vi "Popup.vi"(8 "error in (no error)":errorcluster, 9 "Panel":refnum<class "Panel.lvclass">, 10 "String in":string, 11 "String Data Type in":refnum<class "String Data Type.lvclass">) -> (0 "error out":errorcluster, 2 "String out":string, 3 "String Data Type out":refnum<class "String Data Type.lvclass">)   [LabVIEW 2018, in "String Data Type.lvclass"]
uses:
  String Data Type.lvclass
  <vilib>/MGI/Panel Manager/Panel/Panel/Panel.lvclass
  <vilib>/Utility/miscctls.llb/LVSelectionTypeDef.ctl
  String Data Type.lvclass/String Data Type.ctl
panel:
  in  "String":string
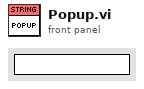
[diagram p1: front panel]
types:
  T1 = typedef "LVSelectionTypeDef.ctl" = cluster{"Selection Start":u32, "Selection End":u32}
  T2 = typedef "String Data Type.lvclass/Display Style Enum.ctl" = enum16{"Normal", "'\\' Codes", "Hex"}
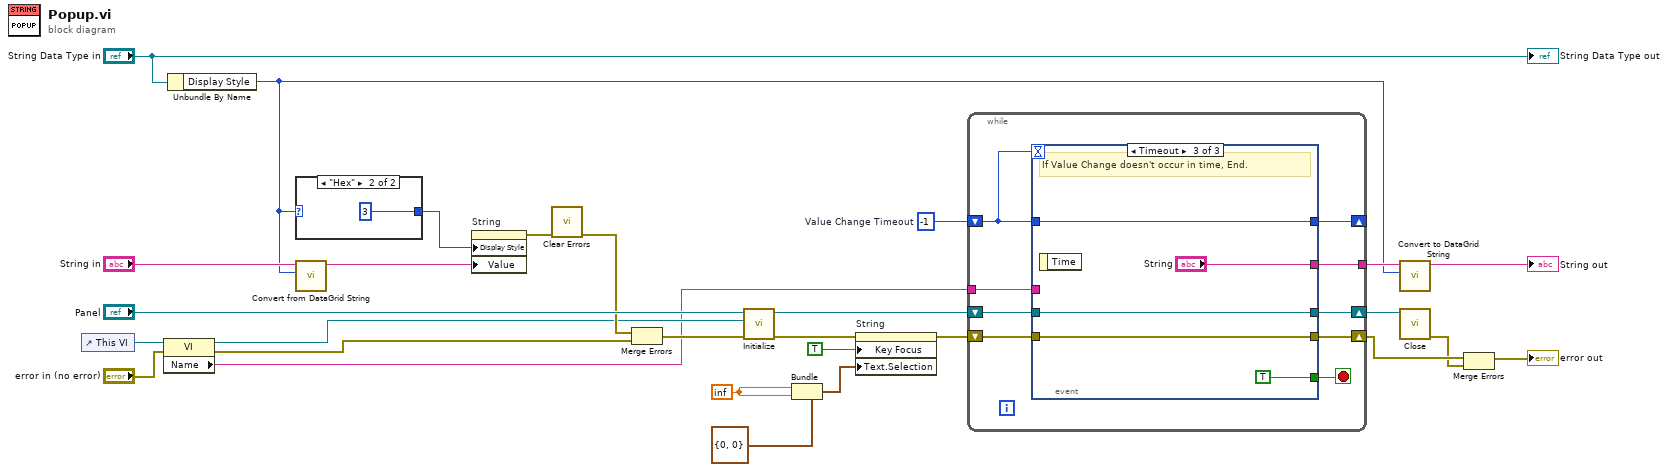
[diagram p0: block diagram]
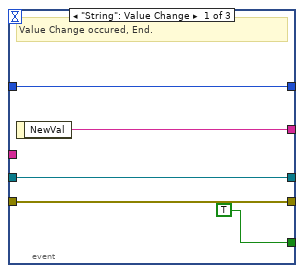
[diagram p3: hidden frame]
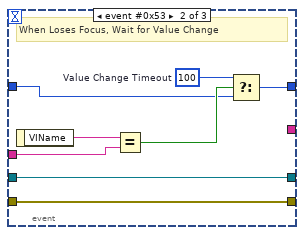
[diagram p4: hidden frame]
diagram:
  w9 = inf
  w14 = -1  # Value Change Timeout
  n1 = control-ref of="This VI"() -> (w20:refnum<vi>)
  n2 = property class="VI"(reference=w20, error in="error in (no error)") -> (reference out=w19:refnum<vi>, error out=w15:errorcluster, "Name"=w17:string)
  n3 = Unbundle By Name("String Data Type in") -> ("Display Style"=w2:T2)
  n4 = case shown="\"Hex\"" w2 {
    selector: w2 -> [w29 _]
    tunnel: [w29 u32 3] -> w1
    frame "Normal", "'\\' Codes" {
    }
    frame "Hex" {
    }
  }
  n5 = call "Convert from DataGrid String.vi"("Display Style"=w2, "DataGrid String in"="String in") -> ("Popup String out"=w6:string)  [unwired: 9 in]
  n6 = property on="String" class="Str"("Display Style"=w1, "Value"=w6) -> (error out=w22:errorcluster)  [unwired: 2 in, 1 out]
  n7 = call <vilib>:"Clear Errors.vi"("error in (no error)"=w22) -> ("error out"=w21:errorcluster)  [unwired: 5 in, 1 out]
  n8 = Merge Errors(w21, w15) -> (w18:errorcluster)
  n9 = call <vilib>:"Initialize.vi"("error in (no error)"=w18, "VI Refnum"=w19, "Panel In"="Panel") -> ("error out"=w12:errorcluster, "Panel Out"=w27:refnum<class "Panel.lvclass">)  [unwired: 6 in, 1 out]
  n10 = Bundle(cluster=T1 {"Selection Start"=0, "Selection End"=0} ("Text.Selection"), "Selection Start"=w9, "Selection End"=w9) -> (w8:T1)
  n11 = property on="String" class="Str"(error in=w12, "Key Focus"=TRUE, "Text.Selection"=w8) -> (error out=w11:errorcluster)  [unwired: 1 in, 1 out]
  n12 = while {
    shift-right: [w39] -> w25
    shift-left: w11 -> [w38]
    shift-right: [w36] -> w26
    shift-left: w27 -> [w35]
    tunnel: [w34] -> w3
    tunnel: w17 -> [w33]
    shift-right: [w31] -> _
    shift-left: w14 -> [w32]
    stop <- w37 stop-if-true
    n13 = event shown="[2] Timeout" {
      selector: _ -> [_ _ _]
      dyn-events: _ -> [_ _ _]
      timeout: w32 -> [_ _ _]
      tunnel: [w41 w50 w55] -> w39
      tunnel: w38 -> [w41 w50 w55]
      tunnel: [TRUE _ TRUE] -> w37
      tunnel: [w43 w49 w56] -> w36
      tunnel: w35 -> [w43 w49 w56]
      tunnel: [w42 _ "String"] -> w34
      tunnel: w33 -> [_ w51 _]
      tunnel: w32 -> [w40 w46 w53]
      tunnel: [w40 w45 w53] -> w31
      event "String": Value Change {
        # "Value Change occured, End."
        n14 = event-data() -> ("NewVal"=w42:string)  [unwired: 1 in]
      }
      event event #0x53 {
        w47 = 100  # Value Change Timeout
        # "When Loses Focus, Wait for Value Change"
        n15 = event-data() -> ("VIName"=w52:string)  [unwired: 1 in]
        n16 = Equal?(x=w52, y=w51) -> (x = y?=w48:bool)
        n17 = Select(t=w47, s=w48, f=w46) -> (s? t:f=w45:i32)
      }
      event Timeout {
        # "If Value Change doesn't occur in time, End."
        n18 = event-data() -> ()  [unwired: 1 in, 1 out]
      }
    }
  }
  n19 = call "Convert to DataGrid String.vi"("Display Style"=w2, "Popup String in"=w3) -> ("DataGrid String out"=→"String out":string)  [unwired: 9 in]
  n20 = call-dynamic "Close.vi"("Panel In"=w26) -> ("Error Out"=w23:errorcluster)  [unwired: 10 in]
  n21 = Merge Errors(w25, w23) -> (→"error out":errorcluster)
  "String Data Type out" <- "String Data Type in"
